vi "Get BLISS_Test Connection.vi"(7 "timeout (10000 ms)":i32=10000 min=1000 max=60000, 8 "error in (no error)":errorcluster, 11 "server":string) -> (0 "error out":errorcluster, 3 "Valid":bool)   [LabVIEW 2020]
uses:
  <vilib>/httpClient/LabVIEWHTTPClient.lvlib
panel:
  out "URL":string
  out "Progress":u8(slide)=1 scale=0.0..100.0
  # "Testing Server Connection ... Please Wait ..."
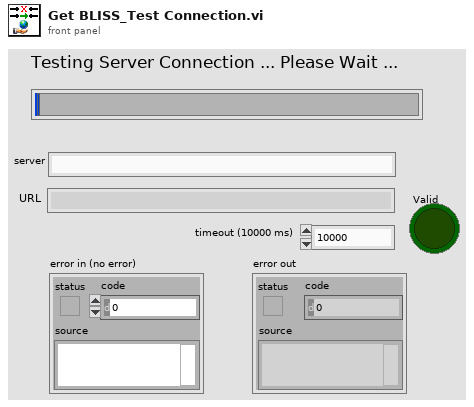
[diagram p1: front panel]
types:
  T1 = typedef "LabVIEWHTTPClient.lvlib/ClientHandle.ctl" = refnum<k1>
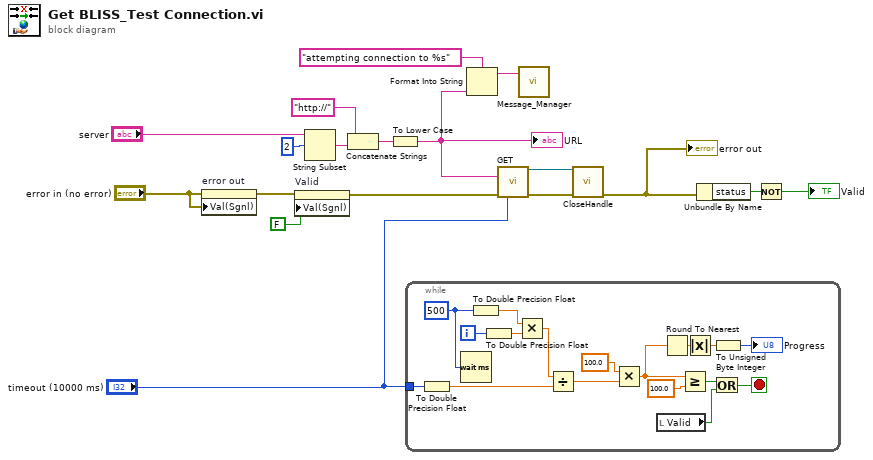
[diagram p0: block diagram]
diagram:
  n1 = property on="error out" class="Clust (strict)"(error in="error in (no error)", "Val(Sgnl)"="error in (no error)") -> (error out=w6:errorcluster)  [unwired: 1 in, 1 out]
  n2 = property on="Valid" class="Bool (strict)"(error in=w6, "Val(Sgnl)"=FALSE ("Value (Signaling)")) -> (error out=w8:errorcluster)  [unwired: 1 in, 1 out]
  n3 = String Subset(string="server", offset (0)=2) -> (substring=w12:string)  [unwired: 1 in]
  n4 = Concatenate Strings("http://" ("string"), w12) -> (w11:string)
  n5 = To Lower Case(string=w11) -> (all lower case string=w17:string)
  "URL" <- w17
  n6 = while {
    tunnel: "timeout (10000 ms)" -> [w32]
    i -> [w34]
    stop <- w26 stop-if-true
    w35 = u32 500 ("milliseconds to wait")
    n7 = To Double Precision Float(number=w32) -> (double precision float=w22:dbl)
    n8 = Wait (ms)(milliseconds to wait=w35) -> ()  [unwired: 1 out]
    n9 = To Double Precision Float(number=w35) -> (double precision float=w23:dbl)
    n10 = To Double Precision Float(number=w34) -> (double precision float=w24:dbl)
    n11 = Multiply(x=w23, y=w24) -> (x*y=w33:dbl)
    n12 = Divide(x=w33, y=w22) -> (x/y=w31:dbl)
    n13 = Multiply(x=100.0, y=w31) -> (x*y=w29:dbl)
    n14 = local read "Valid"() -> (w25:bool)
    n15 = Round To Nearest(number=w29) -> (nearest integer value=w20:dbl)
    n16 = Greater Or Equal?(x=w29, y=100.0) -> (x >= y?=w27:bool)
    n17 = Absolute Value(x=w20) -> (abs(x)=w19:dbl)
    n18 = Or(x=w27, y=w25) -> (x .or. y?=w26:bool)
    n19 = To Unsigned Byte Integer(number=w19) -> (unsigned 8bit integer=→"Progress":u8)
  }
  n20 = Format Into String(format string="attempting connection to %s", w17) -> (resulting string=w4:string)  [unwired: 2 in, 1 out]
  n21 = call <vilib>:"GET.vi"("url"=w17, "error in (no error)"=w8, "timeout (10000)"="timeout (10000 ms)") -> ("client handle out"=w2:T1, "error out"=w3:errorcluster)  [unwired: 9 in, 2 out]
  n22 = call "Message_Manager.vi"("New Entry"=w4) -> ()  [unwired: 5 in, 6 out]
  n23 = call <vilib>:"CloseHandle.vi"("client handle"=w2, "error in (no error)"=w3) -> ("error out"=w1:errorcluster)  [unwired: 13 in]
  "error out" <- w1
  n24 = Unbundle By Name(w1) -> ("status"=w10:bool)
  n25 = Not(x=w10) -> (.not. x?=→"Valid":bool)
